vi "Mem_Str.vi"(8 "error in (no error)":errorcluster, 11 "dataInfo":T1) -> (0 "error out":errorcluster, 2 "response":string)   [LabVIEW 2019, in "Memory Data Access.lvlib"]
uses:
  Memory Data Access.lvlib
  Typedef/memoryDataBlock.ctl
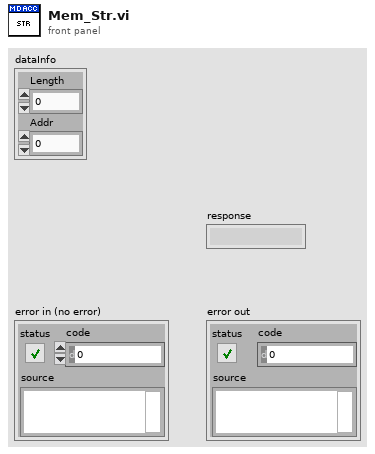
[diagram p1: front panel]
types:
  T1 = typedef "Memory Data Access.lvlib/memoryDataBlock.ctl" = cluster{"Length":u32, "Addr":u64}
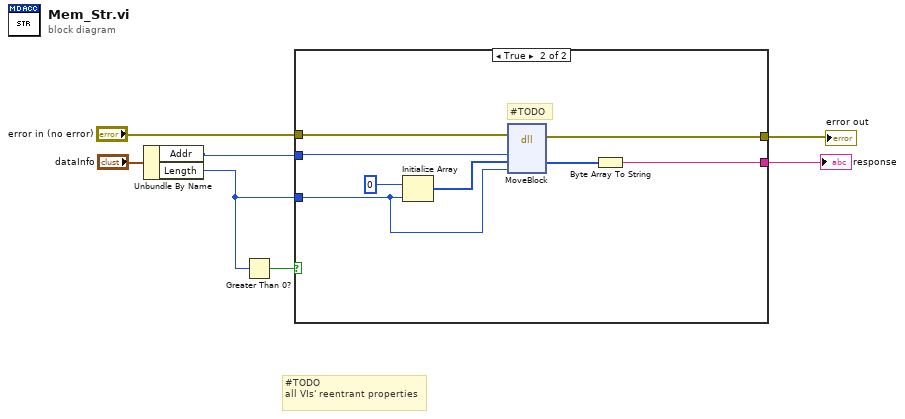
[diagram p0: block diagram]
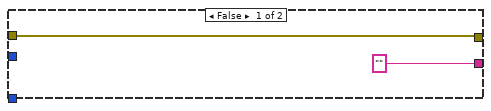
[diagram p2: hidden frame]
diagram:
  # "#TODO\nall VIs' reentrant properties"
  n1 = Unbundle By Name("dataInfo") -> ("Addr"=w2:u64, "Length"=w1:u32)
  n2 = Greater Than 0?(x=w1) -> (x > 0?=w5:bool)
  n3 = case shown="True" w5 {
    tunnel: "error in (no error)" -> [w9 w17]
    tunnel: [w9 w16] -> w6
    tunnel: w2 -> [_ w14]
    tunnel: w1 -> [_ w13]
    tunnel: ["" ("string") w10] -> w4
    frame False {
    }
    frame True {
      # "#TODO"
      n4 = Initialize Array(u8 0, w13) -> (w15:u8[])
      n5 = dll-call lib="LabVIEW" fn="MoveBlock"(error in=w17, "Address"=w14, "Destination"=w15, "Size"=w13) -> (error out=w16:errorcluster, "Destination"=w11:u8[])  [unwired: 5 in, 1 out]
      n6 = Byte Array To String(unsigned byte array=w11) -> (string=w10:string)
    }
  }
  "error out" <- w6
  "response" <- w4
